vi "Test.vi"   [LabVIEW 2017]
doc: "This VI is called when test mode begins, and will automatically be terminated when it ends. You can add manual or automatic tests and invoke them from the dashboard."
uses:
  <vilib>/Rock Robotics/Network Tables/NT Write Numeric Array.vi
  <vilib>/Rock Robotics/Network Tables/NT Write Boolean Array.vi
  <vilib>/Rock Robotics/Network Tables/NT Write Boolean.vi
types:
  T1 = typedef "WPI_RobotDriveDevRef.ctl" = cluster{"DevStatus":errorcluster, "Motors[]":T2[], "Square Inputs":bool, "Max Output":dbl}
  T2 = typedef "WPI_MotorControlDeviceRef.ctl" = cluster{"DeviceStatus":errorcluster, "Type":T3, "PWM":cluster{"PWM Channel":T4, "DeadBand":T5}, "CAN":cluster{"Device Number":u8, "SetOutput VI Ref":variant, "GetOutput VI Ref":variant, "Enable VI Ref":variant, "Disable VI Ref":variant, "Data":variant}, "Invert":bool, "DIO PWM":cluster{"PWM \"Enable\" Channel":T4, "DIOChannel":T6, "PWM Rate":dbl}}
  T3 = typedef "WPI_MotorControlType.ctl" = enum16{"PWM", "CAN", "DIO PWM"}
  T4 = typedef "FPGA_DIOPWMChannel.ctl" = enum8{"PWM 0", "PWM 1", "PWM 2", "PWM 3", "PWM 4", "PWM 5", "PWM 6", "PWM 7", "PWM 8", "PWM 9", "PWM MXP 0", "PWM MXP 1", "PWM MXP 2", "PWM MXP 3", "PWM MXP 4", "PWM MXP 5", "PWM MXP 6", "PWM MXP 7", "PWM MXP 8", "PWM MXP 9", "Invalid"}
  T5 = typedef "WPI_PWMDeadband.ctl" = cluster{"Name":string, "maxPositivePwm":i32, "minPositivePwm":i32, "centerPwm":i32, "maxNegativePwm":i32, "minNegativePwm":i32, "angularRange":u16}
  T6 = typedef "FPGA_DIOChannel.ctl" = enum8{"DIO 0", "DIO 1", "DIO 2", "DIO 3", "DIO 4", "DIO 5", "DIO 6", "DIO 7", "DIO 8", "DIO 9", "DIO MXP 0", "DIO MXP 1", "DIO MXP 2", "DIO MXP 3", "DIO MXP 4", "DIO MXP 5", "DIO MXP 6", "DIO MXP 7", "DIO MXP 8", "DIO MXP 9", "DIO MXP 10", "DIO MXP 11", "DIO MXP 12", "DIO MXP 13", "DIO MXP 14", "DIO MXP 15", "SPI Port CS1", "SPI Port CS2", "SPI Port CS3", "SPI Port MISO", "SPI Port MOSI", "Invalid"}
  T7 = typedef "WPI_JoystickDevRef.ctl" = cluster{"Device":T8}
  T8 = typedef "WPI_JoystickDeviceEnum.ctl" = enum16{"USB 0", "USB 1", "USB 2", "USB 3", "USB 4", "USB 5"}
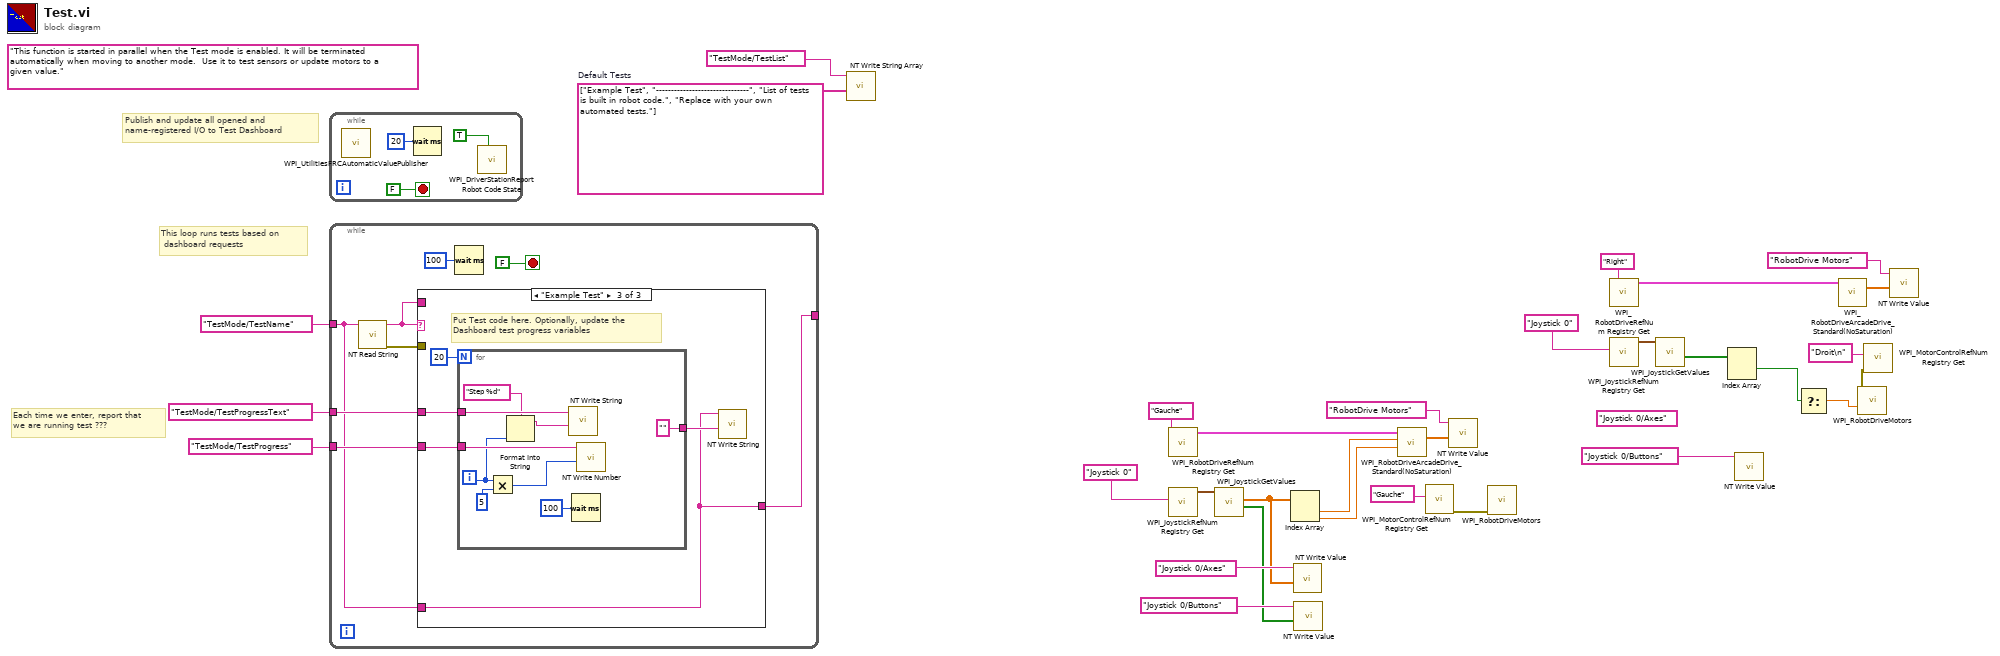
[diagram p0: block diagram]
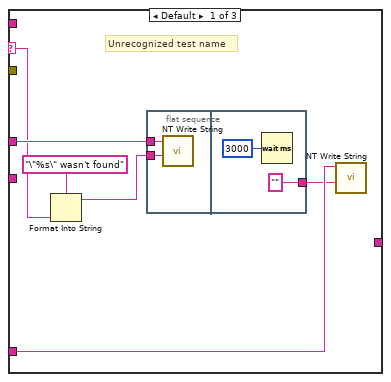
[diagram p2: hidden frame]
diagram:
  (unwired) "Joystick 0/Axes" ("Name")
  w28 = string[] ["Example Test", "-------------------------------", "List of tests is built in robot code.", "Replace with your own automated tests."]  # Default Tests
  (unwired) "This function is started in parallel when the Test mode is enabled. It will be terminated automatically when moving to another mode.  Use it to test sensors or update motors to a given value."
  # "This loop runs tests based on \n dashboard requests"
  # "Publish and update all opened and\nname-registered I/O to Test Dashboard"
  # "Each time we enter, report that\nwe are running test ???"
  n1 = while {
    stop <- FALSE stop-if-true
    n2 = call <vilib>:"WPI_UtilitiesFRCAutomaticValuePublisher.vi"() -> ()  [unwired: 12 in]
    n3 = Wait (ms)(milliseconds to wait=u32 20) -> ()  [unwired: 1 out]
    n4 = call <vilib>:"WPI_DriverStationReport Robot Code State.vi"("Test"=TRUE ("Autonomous")) -> ()  [unwired: 10 in, 1 out]
  }
  n5 = while {
    tunnel: "TestMode/TestName" ("Name") -> [w37]
    tunnel: "TestMode/TestProgressText" ("Name") -> [w40]
    tunnel: "TestMode/TestProgress" ("Name") -> [w39]
    tunnel: [w35] -> _
    stop <- FALSE stop-if-true
    n6 = call <vilib>:"NT Read String.vi"("Name"=w37) -> ("error out"=w36:errorcluster, "String"=w38:string)  [unwired: 9 in]
    n7 = case shown="\"Example Test\"" w38 {
      selector: w38 -> [w47 _ _]
      tunnel: w37 -> [w44 _ w53]
      tunnel: w40 -> [w48 _ w56]
      tunnel: w39 -> [_ _ w57]
      tunnel: w38 -> [_ _ _]
      tunnel: w36 -> [_ _ _]
      tunnel: [_ _ w53] -> w35
      frame Default {
        # "Unrecognized test name"
        n8 = Format Into String(format string="\"%s\" wasn't found" ("Name"), w47) -> (resulting string=w46:string)  [unwired: 2 in, 1 out]
        n9 = flat-sequence {
          tunnel: w48 -> [w49]
          tunnel: w46 -> [w50]
          tunnel: ["" ("Name")] -> w43
          frame #0 {
            n10 = call <vilib>:"NT Write String.vi"("String"=w50, "Name"=w49) -> ()  [unwired: 9 in, 1 out]
          }
          frame #1 {
            n11 = Wait (ms)(milliseconds to wait=u32 3000) -> ()  [unwired: 1 out]
          }
        }
        n12 = call <vilib>:"NT Write String.vi"("String"=w43, "Name"=w44) -> ()  [unwired: 9 in, 1 out]
      }
      frame "" {
        # "No test to run"
      }
      frame "Example Test" {
        # "Put Test code here. Optionally, update the\nDashboard test progress variables"
        n13 = for {
          N: 20 -> [_]
          tunnel: w57 -> [w66]
          tunnel: w56 -> [w64]
          tunnel: ["" ("String")] -> w54
          i -> [w61]
          n14 = Multiply(x=w61, y=u32 5 ("milliseconds to wait")) -> (x*y=w62:u32)
          n15 = Format Into String(format string="Step %d", w61) -> (resulting string=w59:string)  [unwired: 2 in, 1 out]
          n16 = call <vilib>:"NT Write String.vi"("String"=w59, "Name"=w64) -> ()  [unwired: 9 in, 1 out]
          n17 = Wait (ms)(milliseconds to wait=u32 100) -> ()  [unwired: 1 out]
          n18 = call <vilib>:"NT Write Number.vi"("Numeric"=w62, "Name"=w66) -> ()  [unwired: 9 in, 1 out]
        }
        n19 = call <vilib>:"NT Write String.vi"("String"=w54, "Name"=w53) -> ()  [unwired: 9 in, 1 out]
      }
    }
    n20 = Wait (ms)(milliseconds to wait=u32 100) -> ()  [unwired: 1 out]
  }
  n21 = call <vilib>:"NT Write String Array.vi"("String Array"=w28, "Name"="TestMode/TestList") -> ()  [unwired: 9 in, 1 out]
  n22 = call <vilib>:"WPI_RobotDriveRefNum Registry Get.vi"("refnum name"="Gauche") -> ("RobotDriveDevRef"=w21:T1)  [unwired: 1 in, 9 out]
  n23 = call <vilib>:"WPI_JoystickRefNum Registry Get.vi"("refnum name"="Joystick 0") -> ("JoystickDevRef"=w18:T7)  [unwired: 1 in, 9 out]
  n24 = call <vilib>:"WPI_JoystickGetValues.vi"("JoystickDevRef"=w18) -> ("Buttons"=w13:bool[], "Axes"=w14:dbl[])  [unwired: 6 in, 3 out]
  n25 = Index Array(array=w14) -> (element #1=w20:dbl, element #2=w17:dbl)  [unwired: 2 in]
  n26 = call-poly <vilib>:"NT Write Value.vi"("Numeric Array"=w14, "Name"="Joystick 0/Axes") -> ()  [unwired: 9 in, 1 out]
  n27 = call-poly <vilib>:"NT Write Value.vi"("Boolean Array"=w13, "Name"="Joystick 0/Buttons") -> ()  [unwired: 9 in, 1 out]
  n28 = call <vilib>:"WPI_RobotDriveArcadeDrive_Standard(NoSaturation).vi"("Y axis value"=w17, "X axis value"=w20, "RobotDriveDevRef"=w21) -> ("Motor Values"=w12:dbl[])  [unwired: 1 in, 7 out]
  n29 = call <vilib>:"WPI_MotorControlRefNum Registry Get.vi"("refnum name"="Gauche") -> ("error out"=w26:errorcluster)  [unwired: 9 in, 1 out]
  n30 = call-poly <vilib>:"NT Write Value.vi"("Numeric Array"=w12, "Name"="RobotDrive Motors") -> ()  [unwired: 9 in, 1 out]
  n31 = call <vilib>:"WPI_RobotDriveMotors.vi"("error in (no error)"=w26) -> ()  [unwired: 8 in, 3 out]
  n32 = call <vilib>:"WPI_RobotDriveRefNum Registry Get.vi"("refnum name"="Right") -> ("RobotDriveDevRef"=w9:T1)  [unwired: 1 in, 9 out]
  n33 = call <vilib>:"WPI_JoystickRefNum Registry Get.vi"("refnum name"="Joystick 0") -> ("JoystickDevRef"=w7:T7)  [unwired: 1 in, 9 out]
  n34 = call <vilib>:"WPI_JoystickGetValues.vi"("JoystickDevRef"=w7) -> ("Buttons"=w3:bool[])  [unwired: 6 in, 4 out]
  n35 = Index Array(array=w3) -> (element #1=w2:bool)  [unwired: 2 in, 1 out]
  n36 = call-poly <vilib>:"NT Write Value.vi"("Name"="Joystick 0/Buttons") -> ()  [unwired: 10 in, 1 out]
  n37 = Select(s=w2) -> (s? t:f=w1:dbl)  [unwired: 2 in]
  n38 = call <vilib>:"WPI_RobotDriveArcadeDrive_Standard(NoSaturation).vi"("RobotDriveDevRef"=w9) -> ("Motor Values"=w5:dbl[])  [unwired: 3 in, 7 out]
  n39 = call <vilib>:"WPI_MotorControlRefNum Registry Get.vi"("refnum name"="Droit\n") -> ("error out"=w24:errorcluster)  [unwired: 9 in, 1 out]
  n40 = call <vilib>:"WPI_RobotDriveMotors.vi"("error in (no error)"=w24, "RightSpeed"=w1) -> ()  [unwired: 7 in, 3 out]
  n41 = call-poly <vilib>:"NT Write Value.vi"("Numeric Array"=w5, "Name"="RobotDrive Motors") -> ()  [unwired: 9 in, 1 out]
